vi "2-norm of Vector.vi"(11 "V":cdb[](array[numeric])) -> (3 "2-norm of V":dbl)   [LabVIEW 2017, in "NI_AALPro.lvlib"]
uses:
  NI_AALPro.lvlib
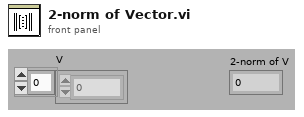
[diagram p1: front panel]
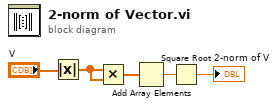
[diagram p0: block diagram]
diagram:
  n1 = Absolute Value(x="V") -> (abs(x)=w4:dbl[])
  n2 = Multiply(x=w4, y=w4) -> (x*y=w3:dbl[])
  n3 = Add Array Elements(numeric array=w3) -> (sum=w2:dbl)
  n4 = Square Root(x=w2) -> (sqrt(x)=→"2-norm of V":dbl)
